vi "filter -- window span logic.vi"(4 "action for \"above\"":T1=enum."shrink", 6 "action for \"below\"":T1=enum."grow", 8 "tale of three indices -- int -- control out":T2={"left"=0, "center"=0, "right"=0, "right most"=0, "left most"=0, "window"=0, "max win factor"=2, "max win"=2, "min win"=2}, 9 "start":bool, 11 "new state":T3) -> (0 "three indices out":T2={"left"=0, "center"=0, "right"=0, "right most"=0, "left most"=0, "window"=0, "max win factor"=2, "max win"=2, "min win"=2}, 1 "stop":bool)   [LabVIEW 2018]
uses:
  tale of three indices -- selector -- control.ctl
  comparison control.ctl
  tale of three indices -- int -- control.ctl
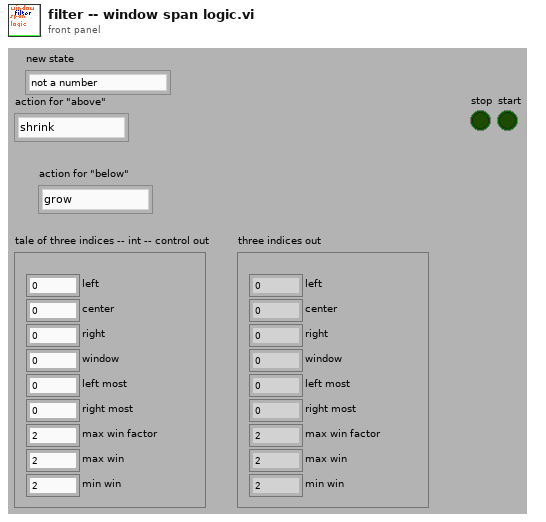
[diagram p1: front panel]
types:
  T1 = typedef "tale of three indices -- selector -- control.ctl" = enum16{"window right", "window left", "balance", "shrink", "grow", "do nothing", "reset", "center right", "center left", "all left", "all right", "right wing shrink", "left wing shrink", "left wing grow", "right wing grow", "skew left", "skew right", "check"}
  T2 = typedef "tale of three indices -- int -- control.ctl" = cluster{"left":i32, "center":i32, "right":i32, "right most":i32, "left most":i32, "window":i32, "max win factor":i32, "max win":i32, "min win":i32}
  T3 = typedef "comparison control.ctl" = enum16{"not a number", "above", "in range", "below"}
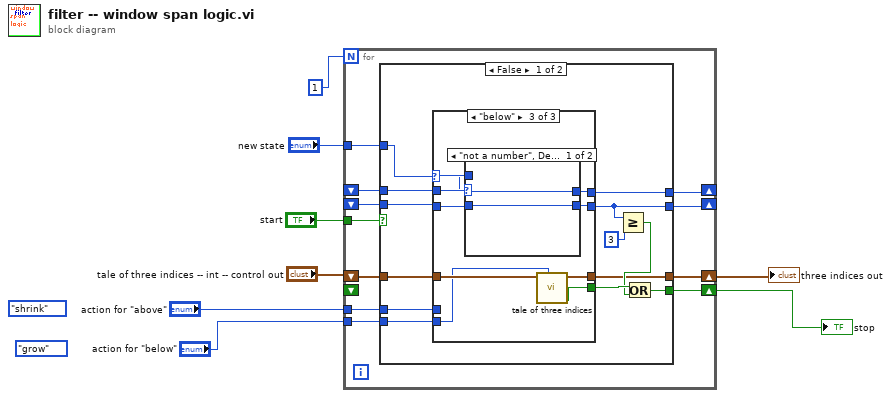
[diagram p0: block diagram]
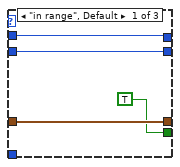
[diagram p2: hidden frame]
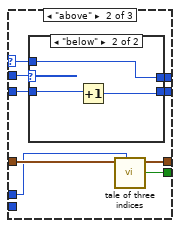
[diagram p3: hidden frame]
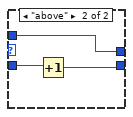
[diagram p5: hidden frame]
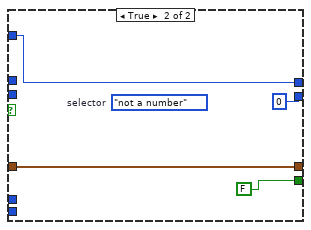
[diagram p6: hidden frame]
diagram:
  (unwired) tale_of_three_indices_--_selector_--_control."grow" ("selector")
  (unwired) tale_of_three_indices_--_selector_--_control."shrink" ("selector")
  n1 = for {
    N: 1 -> [_]
    shift-right: [w17] -> _
    shift-left: _ -> [w16]
    shift-right: [w15] -> _
    shift-left: _ -> [w18]
    shift-right: [w14] -> w7
    shift-left: "tale of three indices -- int -- control out" -> [w13]
    shift-right: [w12] -> w6
    shift-left: _ -> [_]
    tunnel: "start" -> [w11]
    tunnel: "new state" -> [w19]
    tunnel: "action for \"above\"" -> [w10]
    tunnel: "action for \"below\"" -> [w9]
    n2 = case shown="False" w11 {
      tunnel: w19 -> [w29 w65]
      tunnel: w18 -> [w28 _]
      tunnel: [w27 0] -> w17
      tunnel: w16 -> [w26 _]
      tunnel: [w25 w65] -> w15
      tunnel: [w24 w67] -> w14
      tunnel: w13 -> [w23 w67]
      tunnel: [w22 FALSE] -> w12
      tunnel: w10 -> [w21 _]
      tunnel: w9 -> [w20 _]
      frame False {
        n3 = case shown="\"below\"" w29 {
          selector: w29 -> [_ w39 w53]
          tunnel: [TRUE w38 w52] -> w31
          tunnel: [w36 w44 w58] -> w24
          tunnel: w23 -> [w36 w45 w59]
          tunnel: w28 -> [w34 w43 w57]
          tunnel: [w33 w42 w55] -> w27
          tunnel: w26 -> [w33 w41 w56]
          tunnel: [w34 w40 w54] -> w25
          tunnel: w21 -> [_ w37 _]
          tunnel: w20 -> [_ _ w51]
          frame "in range", Default {
          }
          frame "above" {
            n4 = case shown="\"below\"" w43 {
              tunnel: [w46 w48] -> w42
              tunnel: w41 -> [w46 w49]
              tunnel: [w47 w50] -> w40
              tunnel: w39 -> [w47 w50]
              frame "not a number", Default {
              }
              frame "below" {
                n5 = Increment(x=w49) -> (x+1=w48:i32)
              }
            }
            n6 = call "tale of three indices.vi"("selector"=w37, "tale of three indices -- int -- control"=w45) -> ("no success ?"=w38:bool, "tale of three indices -- int -- control out"=w44:T2)  [unwired: 6 in, 2 out]
          }
          frame "below" {
            n7 = case shown="\"not a number\", Default" w57 {
              tunnel: [w60 w62] -> w55
              tunnel: w56 -> [w60 w63]
              tunnel: [w61 w64] -> w54
              tunnel: w53 -> [w61 w64]
              frame "not a number", Default {
              }
              frame "above" {
                n8 = Increment(x=w63) -> (x+1=w62:i32)
              }
            }
            n9 = call "tale of three indices.vi"("selector"=w51, "tale of three indices -- int -- control"=w59) -> ("no success ?"=w52:bool, "tale of three indices -- int -- control out"=w58:T2)  [unwired: 6 in, 2 out]
          }
        }
        n10 = Greater Or Equal?(x=w27, y=3) -> (x >= y?=w30:bool)
        n11 = Or(x=w31, y=w30) -> (x .or. y?=w22:bool)
      }
      frame True {
        (unwired) comparison_control."not a number"  # selector
      }
    }
  }
  "three indices out" <- w7
  "stop" <- w6
